vi "Visa Close_v2_230202-WilliamSchei-PC.vi"(8 "error in (no error)":errorcluster, 11 "ControlBoard VISA":refnum<visa-resource-name>="ControlBoard") -> (0 "error out":errorcluster)   [LabVIEW 2022 SP3]
doc: "This VI will close the Control Board VISA session"
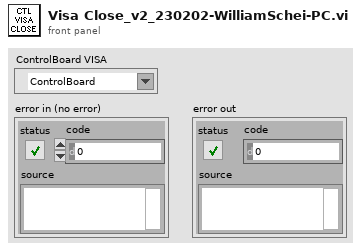
[diagram p1: front panel]
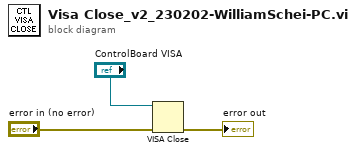
[diagram p0: block diagram]
diagram:
  n1 = VISA Close(VISA resource name="ControlBoard VISA", error in (no error)="error in (no error)") -> (error out=→"error out":errorcluster)
